vi "Get_RESTful_Data.vi"(8 "error in (no error)":errorcluster, 11 "Class in":refnum<class "AB_RESTfulWebService.lvclass">) -> (0 "error out":errorcluster, 2 "data":T1, 3 "Class out":refnum<class "AB_RESTfulWebService.lvclass">)   [LabVIEW 2020, in "AB_RESTfulWebService.lvclass"]
uses:
  <vilib>/AppBuilder/AB_Classes/RESTful/AB_RESTfulWebService.lvclass
  <vilib>/AppBuilder/AB_Classes/RESTful/AB_RESTfulWebService.ctl
  <vilib>/AppBuilder/AB_Classes/RESTful/AB_RESTful_RoutingTemplate.ctl
  <vilib>/AppBuilder/AB_Classes/RESTful/AB_RESTful_RoutingType.ctl
  <vilib>/AppBuilder/AB_Classes/RESTful/AB_RESTful_HTTPMethodType.ctl
  <vilib>/AppBuilder/AB_Classes/RESTful/AB_RESTful_ServiceAttribute.ctl
  <vilib>/AppBuilder/AB_Classes/RESTful/AB_RESTful_ServiceAttributeType.ctl
  <vilib>/AppBuilder/AB_Classes/RESTful/AB_RESTfulWebService.lvclass/AB_RESTfulWebService.ctl
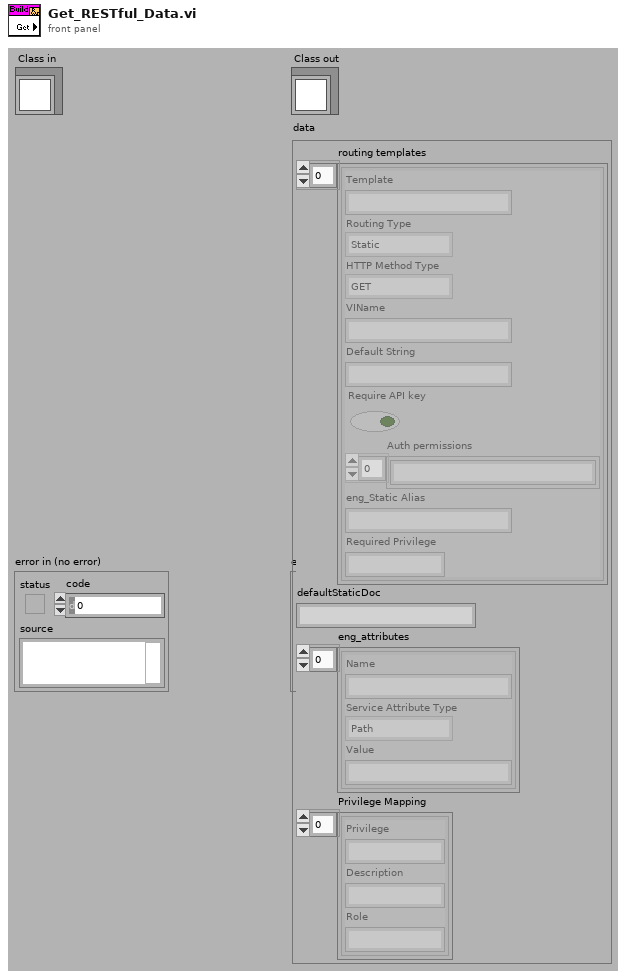
[diagram p1: front panel]
types:
  T1 = typedef "AB_RESTfulWebService.ctl" = cluster{"routing templates":T2[], "defaultStaticDoc":string, "eng_attributes":T5[], "Privilege Mapping":cluster{"Privilege":string, "Description":string, "Role":string}[]}
  T2 = typedef "AB_RESTful_RoutingTemplate.ctl" = cluster{"Template":string, "Routing Type":T3, "HTTP Method Type":T4, "VIName":string, "Default String":string, "Require API key":bool, "Auth permissions":string[], "eng_Static Alias":string, "Required Privilege":string}
  T3 = typedef "AB_RESTful_RoutingType.ctl" = enum32{"Method", "Static"}
  T4 = typedef "AB_RESTful_HTTPMethodType.ctl" = enum32{"GET", "POST", "PUT", "DELETE"}
  T5 = typedef "AB_RESTful_ServiceAttribute.ctl" = cluster{"Name":string, "Service Attribute Type":T6, "Value":string}
  T6 = typedef "AB_RESTful_ServiceAttributeType.ctl" = enum32{"String", "Path"}
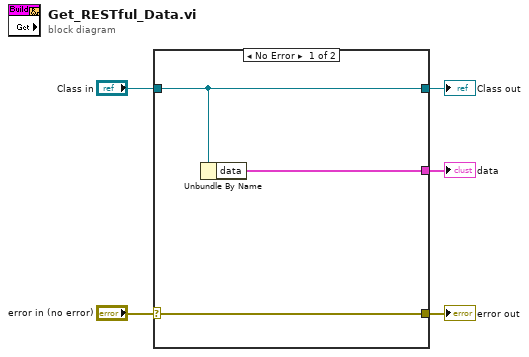
[diagram p0: block diagram]
diagram:
  n1 = case shown="No Error" "error in (no error)" {
    selector: "error in (no error)" -> [w8 w10]
    tunnel: [w8 w10] -> w4
    tunnel: [w7 w9] -> w2
    tunnel: "Class in" -> [w7 w9]
    tunnel: [w6 _] -> w1
    frame No Error {
      n2 = Unbundle By Name(w7) -> ("data"=w6:T1)
    }
    frame Error {
    }
  }
  "Class out" <- w2
  "error out" <- w4
  "data" <- w1
